vi "TSPopup.Update Cell String.vi"(8 "error in (no error)":errorcluster, 9 "Call Data (must be Cell Info cluster)":variant, 11 "Popup Value":variant) -> (0 "error out":errorcluster)   [LabVIEW 2013]
doc: "Changes the text of the location that was clicked on to reflect whatever is contained in <B>Popup Value</B>. This subVI must be used in the <Popup Event> event, which provides the needed inputs.\n<B>NOTE</B> : This only works if the Cell Info cluster was used directly as the Call Data.\n\n<B>Popup Value</B> - Value entered into the Type Sensitive Popup.\n<B>Call data</B> - Call data returned by <Popup Event> event (must be the Cell Info cluster).\n\nType Sensitive Popup \nCopyright © 2007, J. David Saunders\nAll rights reserved."
uses:
  TSPopup.Grid.Cell Info.ctl
  TSPopup.Data Type.ctl
panel:
  in  "rect":T1
  in  "point":cluster{"x":i16, "y":i16}
  in  "Cell Info (type only)":T2
  # "Type Sensitive Popup \nCopyright © 2007, J. David Saunders\nAll rights reserved."
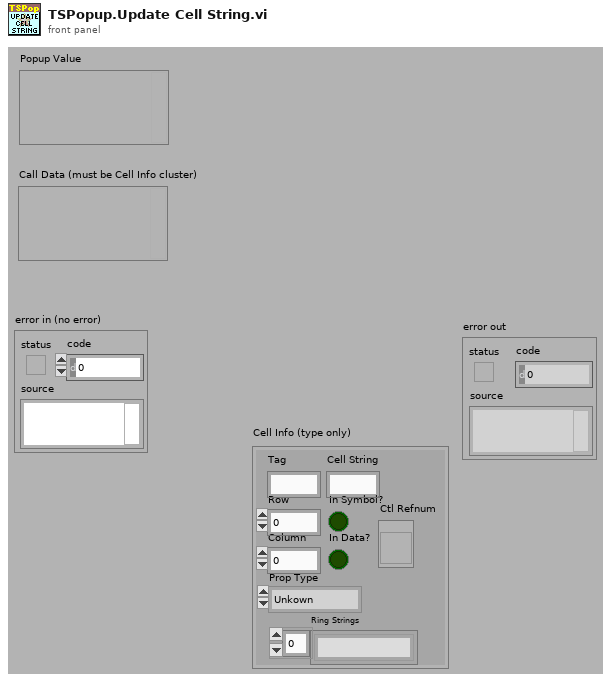
[diagram p1: front panel]
types:
  T1 = cluster{"left":i16, "top":i16, "right":i16, "bottom":i16}
  T2 = typedef "TSPopup.Grid.Cell Info.ctl" = cluster{"Tag":string, "Row":i32, "Column":i32, "In Symbol?":bool, "In Data?":bool, "Cell String":string, "Ctl Refnum":refnum<vi>, "Prop Type":T3, "Ring Strings":string[]}
  T3 = typedef "TSPopup.Data Type.ctl" = enum16{"Unkown", "NO POPUP", "String", "Integer", "Float", "Color", "Boolean", "Ring", "Captioned String", "Captioned Integer", "Button Color", "2 Int Cluster", "4 Int Cluster"}
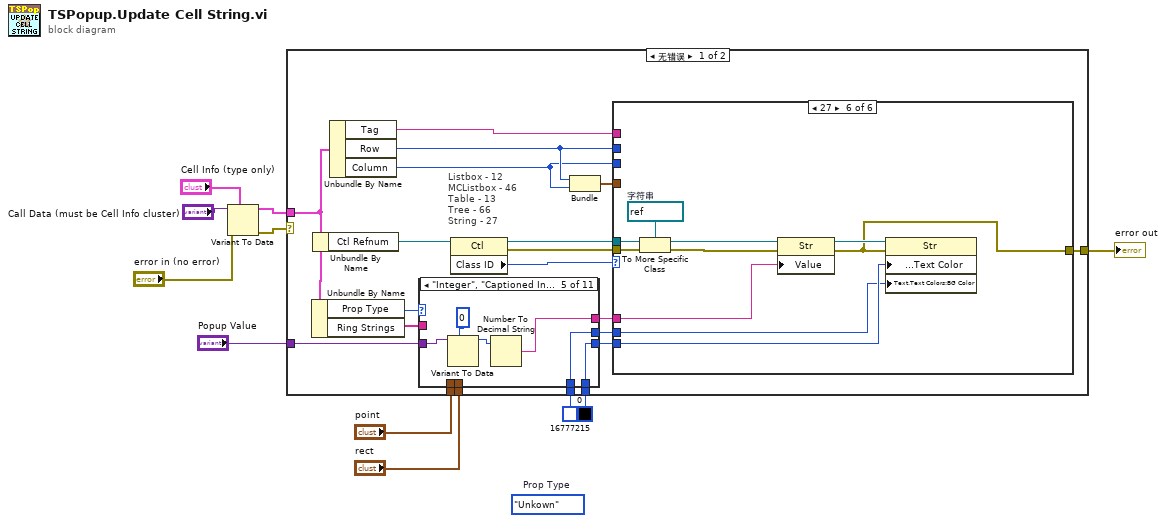
[diagram p0: block diagram]
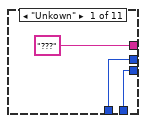
[diagram p2: hidden frame]
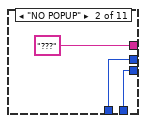
[diagram p3: hidden frame]
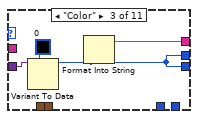
[diagram p4: hidden frame]
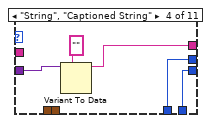
[diagram p5: hidden frame]
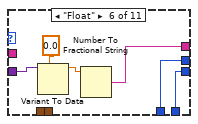
[diagram p6: hidden frame]
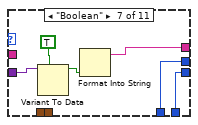
[diagram p7: hidden frame]
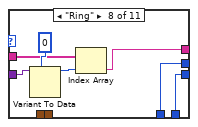
[diagram p8: hidden frame]
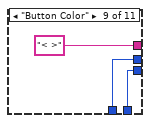
[diagram p9: hidden frame]
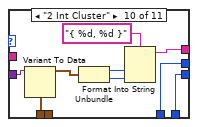
[diagram p10: hidden frame]
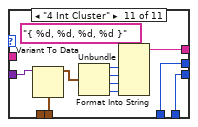
[diagram p11: hidden frame]
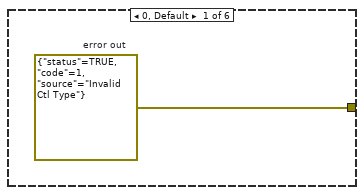
[diagram p12: hidden frame]
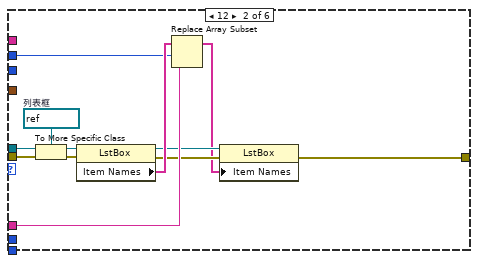
[diagram p13: hidden frame]
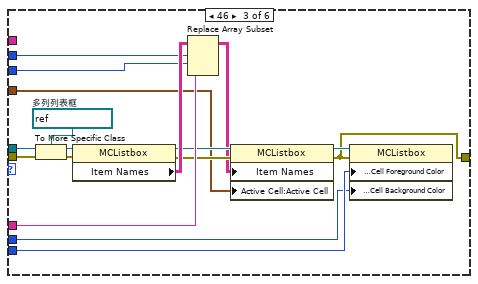
[diagram p14: hidden frame]
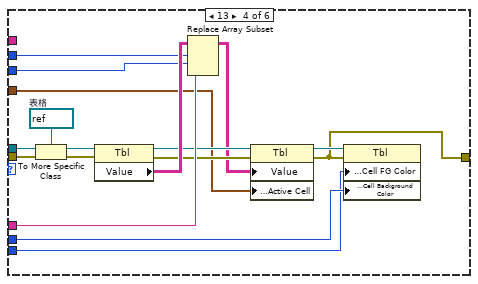
[diagram p15: hidden frame]
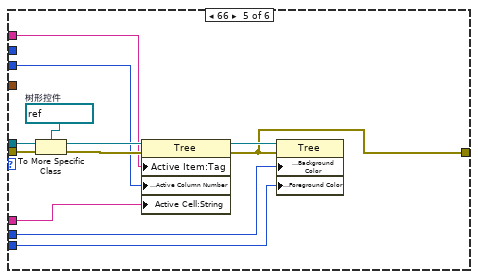
[diagram p16: hidden frame]
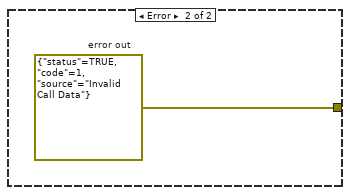
[diagram p17: hidden frame]
diagram:
  (unwired) TSPopup.Data_Type."Unkown"  # Prop Type
  n1 = Variant To Data(error in="error in (no error)", type="Cell Info (type only)", Variant="Call Data (must be Cell Info cluster)") -> (data=w9:T2, error out=w7:errorcluster)
  n2 = case shown="无错误" w7 {
    tunnel: w9 -> [w25 _]
    tunnel: [w26 w164] -> w8
    tunnel: "Popup Value" -> [w23 _]
    tunnel: "point" -> [w21 _]
    tunnel: "rect" -> [w20 _]
    tunnel: u32 0 -> [w16 _]
    tunnel: u32 16777215 -> [w15 _]
    frame No Error {
      # "Listbox - 12\nMCListbox - 46\nTable - 13\nTree - 66\nString - 27"
      n3 = Unbundle By Name(w25) -> ("Prop Type"=w19:T3, "Ring Strings"=w24:string[])
      n4 = Unbundle By Name(w25) -> ("Ctl Refnum"=w28:refnum<vi>)
      n5 = Unbundle By Name(w25) -> ("Tag"=w27:string, "Row"=w14:i32, "Column"=w13:i32)
      n6 = case shown="\"Integer\", \"Captioned Integer\"" w19 {
        tunnel: w24 -> [_ _ _ _ _ _ _ w69 _ _ _]
        tunnel: w23 -> [_ _ w41 w43 w50 w56 w62 w71 _ w83 w94]
        tunnel: ["???" "???" w39 w42 w47 w53 w59 w67 "< >" w77 w90] -> w22
        tunnel: w21 -> [_ _ _ _ _ _ _ _ _ w82 _]
        tunnel: w20 -> [_ _ _ _ _ _ _ _ _ _ w89]
        tunnel: [w32 w35 w38 w46 w52 w58 w64 w65 w72 w76 w85] -> w18
        tunnel: [w33 w36 w38 w45 w51 w57 w63 w66 w73 w75 w84] -> w17
        tunnel: w16 -> [w32 w35 _ w46 w52 w58 w64 w65 w72 w76 w85]
        tunnel: w15 -> [w33 w36 _ w45 w51 w57 w63 w66 w73 w75 w84]
        frame "Unkown" {
        }
        frame "NO POPUP" {
        }
        frame "Color" {
          n7 = Variant To Data(type=u32 0, Variant=w41) -> (data=w38:u32)  [unwired: 1 in, 1 out]
          n8 = Format Into String(w38) -> (resulting string=w39:string)  [unwired: 3 in, 1 out]
        }
        frame "String", "Captioned String" {
          n9 = Variant To Data(type="", Variant=w43) -> (data=w42:string)  [unwired: 1 in, 1 out]
        }
        frame "Integer", "Captioned Integer" {
          n10 = Variant To Data(type=0, Variant=w50) -> (data=w48:i32)  [unwired: 1 in, 1 out]
          n11 = Number To Decimal String(number=w48) -> (decimal integer string=w47:string)  [unwired: 1 in]
        }
        frame "Float" {
          n12 = Variant To Data(type=0.0, Variant=w56) -> (data=w54:dbl)  [unwired: 1 in, 1 out]
          n13 = Number To Fractional String(number=w54) -> (F-format string=w53:string)  [unwired: 3 in]
        }
        frame "Boolean" {
          n14 = Variant To Data(type=TRUE, Variant=w62) -> (data=w60:bool)  [unwired: 1 in, 1 out]
          n15 = Format Into String(w60) -> (resulting string=w59:string)  [unwired: 3 in, 1 out]
        }
        frame "Ring" {
          n16 = Variant To Data(type=0, Variant=w71) -> (data=w68:i32)  [unwired: 1 in, 1 out]
          n17 = Index Array(array=w69, index=w68) -> (element=w67:string)
        }
        frame "Button Color" {
        }
        frame "2 Int Cluster" {
          n18 = Variant To Data(type=w82, Variant=w83) -> (data=w78:cluster{"x":i16, "y":i16})  [unwired: 1 in, 1 out]
          n19 = Unbundle(w78) -> ("x"=w80:i16, "y"=w79:i16)
          n20 = Format Into String(format string="{ %d, %d }" ("String"), w80, w79) -> (resulting string=w77:string)  [unwired: 2 in, 1 out]
        }
        frame "4 Int Cluster" {
          n21 = Variant To Data(type=w89, Variant=w94) -> (data=w91:T1)  [unwired: 1 in, 1 out]
          n22 = Unbundle(w91) -> ("left"=w93:i16, "top"=w92:i16, "right"=w88:i16, "bottom"=w87:i16)
          n23 = Format Into String(format string="{ %d, %d, %d, %d }" ("String"), w93, w92, w88, w87) -> (resulting string=w90:string)  [unwired: 2 in, 1 out]
        }
      }
      n24 = property class="Ctl"(reference=w28) -> (reference out=w30:refnum<vi>, error out=w29:errorcluster, "Class ID"=w31:u32)  [unwired: 1 in]
      n25 = Bundle("Row"=w14, "Column"=w13) -> (w12:cluster{"Row":i32, "Column":i32})  [unwired: 1 in]
      n26 = case shown="27" w31 {
        tunnel: w30 -> [_ w106 w123 w140 w152 w162]
        tunnel: w29 -> [_ w105 w122 w139 w151 w161]
        tunnel: w22 -> [_ w101 w118 w135 w146 w158]
        tunnel: w14 -> [_ w97 w114 w131 _ _]
        tunnel: w13 -> [_ _ w113 w130 w147 _]
        tunnel: w27 -> [_ _ _ _ w148 _]
        tunnel: [w95 w96 w108 w125 w142 w154] -> w26
        tunnel: w18 -> [_ _ w110 w126 w144 w156]
        tunnel: w17 -> [_ _ w109 w127 w143 w155]
        tunnel: w12 -> [_ _ w112 w129 _ _]
        frame 0, Default {
          w95 = errorcluster {"status"=TRUE, "code"=1, "source"="Invalid Ctl Type"}  # error out
        }
        frame 12 {
          w107 = refnum<vi> refnum  # 列表框
          n27 = To More Specific Class(target class=w107, reference=w106, error in=w105) -> (specific class reference=w104:refnum<vi>, error out=w103:errorcluster)
          n28 = property class="LstBox"(reference=w104, error in=w103) -> (reference out=w100:refnum<vi>, error out=w99:errorcluster, "Item Names"=w102:string[])
          n29 = Replace Array Subset(array=w102, new element=w101, index=w97) -> (w98:string[])
          n30 = property class="LstBox"(reference=w100, error in=w99, "Item Names"=w98) -> (error out=w96:errorcluster)  [unwired: 1 out]
        }
        frame 46 {
          w124 = refnum<vi> refnum  # 多列列表框
          n31 = To More Specific Class(target class=w124, reference=w123, error in=w122) -> (specific class reference=w121:refnum<vi>, error out=w120:errorcluster)
          n32 = property class="MCListbox"(reference=w121, error in=w120) -> (reference out=w117:refnum<vi>, error out=w116:errorcluster, "Item Names"=w119:string[][])
          n33 = Replace Array Subset(array=w119, new element=w118, index (row)=w114, index (col)=w113) -> (w115:string[][])
          n34 = property class="MCListbox"(reference=w117, error in=w116, "Item Names"=w115, "Active Cell:Active Cell"=w112) -> (reference out=w111:refnum<vi>, error out=w108:errorcluster)
          n35 = property class="MCListbox"(reference=w111, error in=w108, "Active Cell:Cell Foreground Color"=w110, "Active Cell:Cell Background Color"=w109) -> ()  [unwired: 2 out]
        }
        frame 13 {
          w141 = refnum<vi> refnum  # 表格
          n36 = To More Specific Class(target class=w141, reference=w140, error in=w139) -> (specific class reference=w138:refnum<vi>, error out=w137:errorcluster)
          n37 = property class="Tbl"(reference=w138, error in=w137) -> (reference out=w134:refnum<vi>, error out=w133:errorcluster, "Value"=w136:string[][])
          n38 = Replace Array Subset(array=w136, new element=w135, index (row)=w131, index (col)=w130) -> (w132:string[][])
          n39 = property class="Tbl"(reference=w134, error in=w133, "Value"=w132, "Active Cell:Active Cell"=w129) -> (reference out=w128:refnum<vi>, error out=w125:errorcluster)
          n40 = property class="Tbl"(reference=w128, error in=w125, "Active Cell:Cell FG Color"=w126, "Active Cell:Cell Background Color"=w127) -> ()  [unwired: 2 out]
        }
        frame 66 {
          w153 = refnum<vi> refnum  # 树形控件
          n41 = To More Specific Class(target class=w153, reference=w152, error in=w151) -> (specific class reference=w150:refnum<vi>, error out=w149:errorcluster)
          n42 = property class="Tree"(reference=w150, error in=w149, "Active Item:Tag"=w148, "Active Cell:Active Column Number"=w147, "Active Cell:String"=w146) -> (reference out=w145:refnum<vi>, error out=w142:errorcluster)
          n43 = property class="Tree"(reference=w145, error in=w142, "Active Cell:Background Color"=w143, "Active Cell:Foreground Color"=w144) -> ()  [unwired: 2 out]
        }
        frame 27 {
          w163 = refnum<vi> refnum  # 字符串
          n44 = To More Specific Class(target class=w163, reference=w162, error in=w161) -> (specific class reference=w160:refnum<vi>, error out=w159:errorcluster)
          n45 = property class="Str"(reference=w160, error in=w159, "Value"=w158) -> (reference out=w157:refnum<vi>, error out=w154:errorcluster)
          n46 = property class="Str"(reference=w157, error in=w154, "Text.Text Colors:Text Color"=w156, "Text.Text Colors:BG Color"=w155) -> ()  [unwired: 2 out]
        }
      }
    }
    frame Error {
      w164 = errorcluster {"status"=TRUE, "code"=1, "source"="Invalid Call Data"}  # error out
    }
  }
  "error out" <- w8
